vi "FTW-JSON-Object-SetElement.vi"(0 "JSON Object":refnum<class "FTW-JSON.lvclass">, 5 "Key":string, 7 "Value":string, 11 "error in":errorcluster) -> (4 "JSON Object out":refnum<class "FTW-JSON.lvclass">, 15 "error out":errorcluster)   [LabVIEW 2012, in "FTW-JSON.lvclass"]
uses:
  FTW-JSON.lvclass
  FTW-JSON.lvclass/FTW-JSON.ctl
panel:
  # "Inputs"
  # "Outputs"
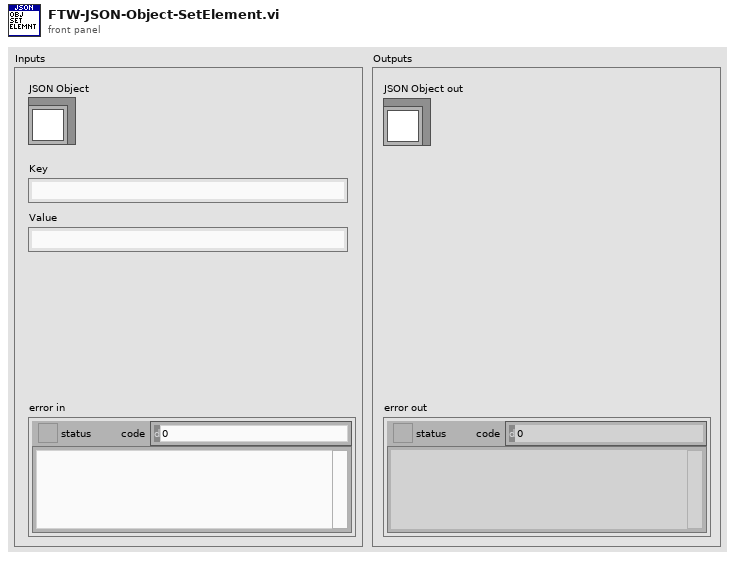
[diagram p1: front panel]
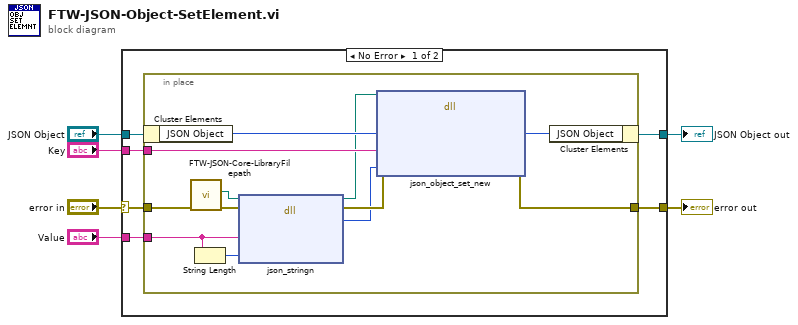
[diagram p0: block diagram]
diagram:
  n1 = case shown="No Error" "error in" {
    selector: "error in" -> [w12 w26]
    tunnel: [w11 w26] -> w6
    tunnel: [w9 w25] -> w4
    tunnel: "JSON Object" -> [w10 w25]
    tunnel: "Key" -> [w8 _]
    tunnel: "Value" -> [w7 _]
    frame No Error {
      n2 = in-place {
        in-place-border: w12 -> [w24]
        in-place-border: [w23] -> w11
        in-place-border: w8 -> [w20]
        in-place-border: w7 -> [w15]
        n3 = in-place-cluster #1(w10) -> ("JSON Object"=w22:i64)
        n4 = call "FTW-JSON-Core-LibraryFilepath.vi"("error in"=w24) -> ("error out"=w17:errorcluster, "JSON Library Filepath"=w19:path)  [unwired: 9 in]
        n5 = String Length(string=w15) -> (length=w14:i32)
        n6 = dll-call lib="?" fn="json_stringn"(path in=w19, error in=w17, "String Value"=w15, "String Length"=w14) -> (path out=w18:path, error out=w16:errorcluster, "New String Value"=w13:i64)  [unwired: 3 in]
        n7 = dll-call lib="?" fn="json_object_set_new"(path in=w18, error in=w16, "JSON Object Pointer"=w22, "Key"=w20, "New JSON Object"=w13) -> (error out=w23:errorcluster, "JSON Object Pointer"=w21:i64)  [unwired: 4 in, 1 out]
        n8 = in-place-cluster #1("JSON Object"=w21) -> (w9:refnum<class "FTW-JSON.lvclass">)
      }
    }
    frame Error {
    }
  }
  "error out" <- w6
  "JSON Object out" <- w4
